vi "Resolve Names.vi"(6 "Error In":errorcluster, 8 "Path In":string, 9 "SystemLin Tag Module configuration":refnum<class "SystemLink configuration.lvclass">) -> (0 "Error Out":errorcluster, 2 "Path Out":string)   [LabVIEW 2015, in "SystemLink runtime.lvclass"]
doc: "Conditionally prepend Minion ID and resolve any template literals."
uses:
  SystemLink runtime.lvclass
  configuration/SystemLink configuration.lvclass
  configuration/SystemLink configuration.lvclass/SystemLink configuration.ctl
  configuration/Read Prepend Minion ID.vi
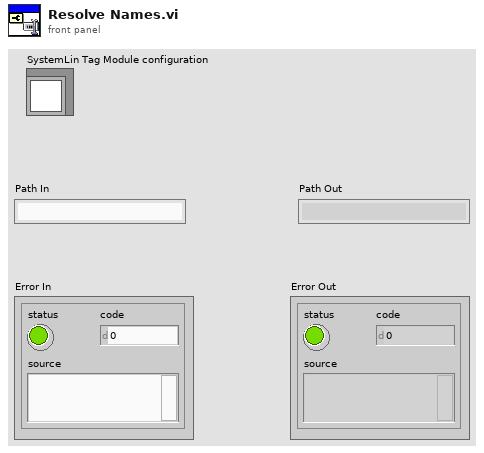
[diagram p1: front panel]
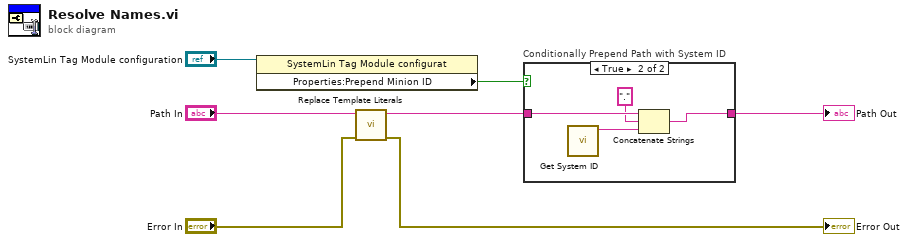
[diagram p0: block diagram]
diagram:
  n1 = property class="SystemLin Tag Module configurat"(reference="SystemLin Tag Module configuration") -> ("Properties:Prepend Minion ID"=w6:bool)  [unwired: 1 in, 2 out]
  n2 = call "Replace Template Literals.vi"("Error In"="Error In", "Path In"="Path In") -> ("Error Out"=→"Error Out":errorcluster, "Path Out"=w1:string)  [unwired: 8 in]
  n3 = case "Conditionally Prepend Path with System ID" shown="True" w6 {
    tunnel: w1 -> [w8 w12]
    tunnel: [w8 w10] -> w5
    frame False {
    }
    frame True {
      # "Prepend with System ID"
      n4 = call "Get System ID.vi"() -> ("SystemID"=w9:string)  [unwired: 11 in]
      n5 = Concatenate Strings(w12, "." ("string"), w9) -> (w10:string)
    }
  }
  "Path Out" <- w5
